vi "Check and Create XML.vi"(8 "Error In":errorcluster, 11 "Path In":path) -> (0 "Error Out":errorcluster, 3 "Path Out":path)   [LabVIEW 2010]
uses:
  Calibration dates.ctl
  <vilib>/Utility/xml.llb/Write to XML File(string).vi
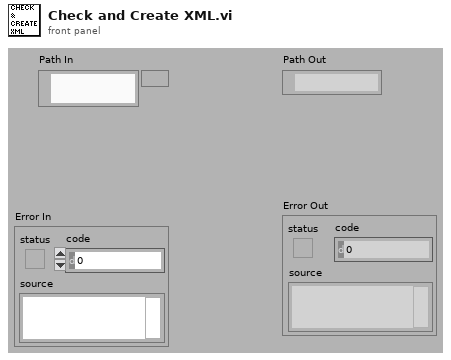
[diagram p1: front panel]
types:
  T1 = typedef "Calibration dates.ctl" = cluster{"Parameter":string, "Last_ST_Date":string, "ST_Due_Date":string, "Corrections":string}
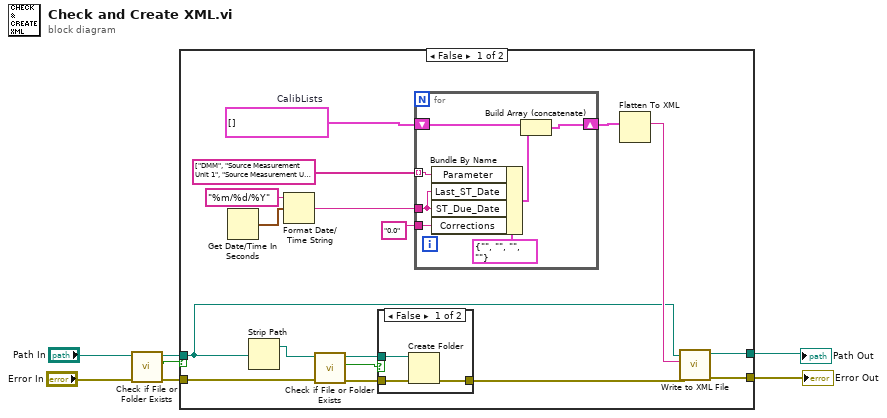
[diagram p0: block diagram]
diagram:
  n1 = call <vilib>:"Check if File or Folder Exists.vi"("error in (no error)"="Error In", "path"="Path In") -> ("error out"=w2:errorcluster, "file or folder exists?"=w6:bool, "dup path"=w5:path)  [unwired: 7 in]
  n2 = case shown="False" w6 {
    tunnel: w5 -> [w14 w37]
    tunnel: [w16 w37] -> w4
    tunnel: w2 -> [w13 w36]
    tunnel: [w15 w36] -> w1
    frame False {
      w19 = T1[] []  # CalibLists
      n3 = Get Date/Time In Seconds() -> (seconds since 1Jan1904=w23:timestamp)
      n4 = Strip Path(path=w14) -> (stripped path=w12:path)  [unwired: 1 out]
      n5 = Format Date/Time String(time format string (%c)="%m/%d/%Y", seconds (now)=w23) -> (date/time string=w21:string)  [unwired: 1 in]
      n6 = call <vilib>:"Check if File or Folder Exists.vi"("error in (no error)"=w13, "path"=w12) -> ("error out"=w11:errorcluster, "file or folder exists?"=w9:bool, "dup path"=w8:path)  [unwired: 7 in]
      n7 = case shown="False" w9 {
        tunnel: w11 -> [w27 w28]
        tunnel: [w26 w28] -> w10
        tunnel: w8 -> [w25 _]
        frame False {
          n8 = Create Folder(path (use dialog)=w25, error in=w27) -> (error out=w26:errorcluster)  [unwired: 1 in, 2 out]
        }
        frame True {
        }
      }
      n9 = for {
        tunnel: string[] ["DMM", "Source Measurement Unit 1", "Source Measurement Unit 2", "Source Measurement Unit 3", "Arbitary waveform Generator", "Digitizer", "Digitizer Prescalar Amplifier", "Counter |timer"] ("Parameter_List") -> [w35] mode=indexing
        tunnel: w21 -> [w34]
        tunnel: "0.0" ("date/time string") -> [w33]
        shift-right: [w30] -> w17
        shift-left: w19 -> [w32]
        n10 = Bundle By Name(cluster=T1 {"Parameter"="", "Last_ST_Date"="", "ST_Due_Date"="", "Corrections"=""} ("Calib_info"), "Parameter"=w35, "Last_ST_Date"=w34, "ST_Due_Date"=w34, "Corrections"=w33) -> (w31:T1)
        n11 = Build Array (concatenate)(w32, w31) -> (w30:T1[])
      }
      n12 = Flatten To XML(anything=w17) -> (xml string=w18:string)
      n13 = call-poly <vilib>:"Write to XML File.vi"("error in (no error)"=w10, "XML Input"=w18, "XML File Path"=w14) -> ("error out"=w15:errorcluster, "XML File Path(duplicate)"=w16:path)  [unwired: 6 in, 1 out]
    }
    frame True {
    }
  }
  "Error Out" <- w1
  "Path Out" <- w4
